vi "AlliGator Launcher.vi"() -> ()   [LabVIEW 2021, in "AlliGator GUI.lvlib"]
doc: "Runs transparently.\nLaunches AlliGator in transparent mode until initialization is complete."
uses:
  AlliGator GUI.lvlib
  AlliGator Variables List.ctl
  Notebook/Notebook Parameters List.ctl
  AlliGator Globals.vi
  AlliGator Check Version.vi
  Variant/Variant to Data/Variant to Boolean.vi
  <userlib>/_OpenG.lib/array/array.llb/Filter 1D Array (String)__ogtk.vi
  AlliGator Globals, Variables & Constants.lvlib
  Variant/Variant to Data/Variant to Data.lvlib
  Notebook/Notebook.lvlib
  Utilities/Utilities.lvlib
  AlliGator Action Engine.lvlib
  Error/Error.lvlib
  <userlib>/_OpenG.lib/array/array.llb/openg_array.lvlib
panel:
  out "About Message":string="© 2015-2023 The Regents of University of California\nAuthor: X. Michalet, Department of Chemistry & Biochemistry, UCLA\n\nThis software product was developed using LabVIEW™ and the National Instruments Vision Development Toolkit for LabVIEW. LabVIEW is a trademark of National Instruments.\n\nFunding was provided in part by grants from the US National Institute of Health, US Department of Energy, UC Cancer Research Coordination Committee and the UCLA Jonsson Comprehensive Cancer Center. AlliGator is not endorsed by, or sponsored by any of the above organizations.\n\nThis software is provided without guaranty of any kind, whether expressed or implied."
  out "Message":string
  out "Version":string
  out "Alligator":string="  AlliGator"
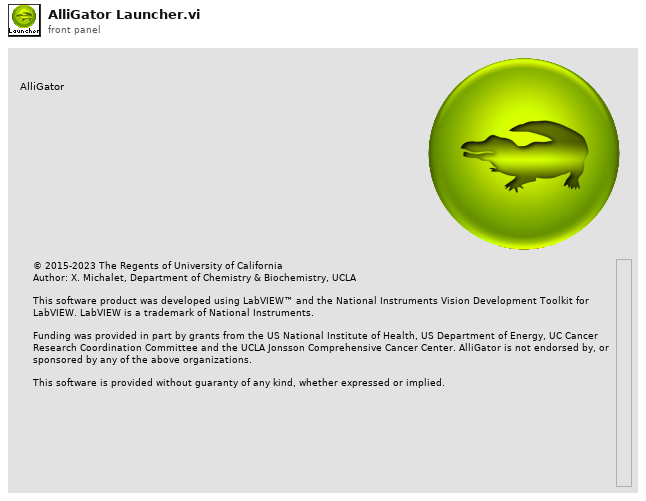
[diagram p1: front panel]
types:
  T1 = typedef "Notebook.lvlib/Notebook Parameters List.ctl" = enum16{"First Opening?", "Saved Notebook?", "Saved Notebook Path", "Beep on Error?"}
  T2 = enum32{"Invalid", "Standard", "Closed", "Hidden", "Minimized", "Maximized"}
  T3 = typedef "AlliGator Globals, Variables & Constants.lvlib/AlliGator Variables List.ctl" = enum16{"---- GUI ----", "Initialization Status", "State Indicators Refnum", "Original AlliGator Menu Items", "Current Action Loop State", "Script in progress", "Playback", "Loop Playback", "Search ROI Used", "Search ROI", "Decay Graph Max Legend Size", "Intensity Graph Max Legend Size", "Decay Statistics Graph Max Legend Size", "Phasor Graph Max Legend Size", "Phasor Ratio Graph Max Legend Size", "Lifetime Graph Max Legend Size", "---- Files ----", "Export Dataset Frames as Individual Files", "Show Batch Export Help Balloons", "Frames in Dataset", "ptu File Frame Start Indices", "Current Frame in Dataset", "Current Frame Timestamp", "------ Python Plugins ------", "Python Plugins Information", "Python Session", "Valid Python Session?", "---- Source Image ----", "Dataset Loaded", "Dataset Metadata", "Dataset Channel", "Dataset Data Description", "Background Dataset Metadata", "Background Dataset Channel", "Background Dataset Data Description", "Background File Subtraction", "Background File Path", "Background File Pile-up Correction", "Background File Pixel Well Capacity", "Background File Scaling Factor", "Source Image ROIs", "Current Source Image ROI", "Source Image ROI Event Refnum", "X_Source Image Display Range", "X_Source Image Palette Information", "Source Image Palette List", "Source Image Scale", "Current Dataset Load Settings", "Source Image:ROI Overlay Color", "---- Image Profile Window ----", "Image Profile:Overlay ROI in Source Image", "Image Profile Window Event Refnum", "Image Profile:IntensityType", "Image Profile:Intensity Average Type", "Image Profile:Intensity-weighted SDV", "Image Profile:Box Profile Type", "Image Profile Window Open", "Image Profile:Plotted Fit Parameter", "X_Type of Displayed Image", "X_Time Gate Slider", "Dataset Path", "Source Image Overlay to Erase", "Is Displayed Image Accumulated", "White Light Image Modified", "Mask Image Modified", "Macrotime Gate Separation", "------ Phasor Graph -------", "Phasor Graph:Show Line", "---- Phasor Plot ---", "Phasor Plot Parameters Changed", "FLI Dataset Modified since last Phasor Plot Calculation", "Phasor Harmonics Data", "Selected Phasor Harmonics", "Phasor Harmonic Manager Event Refnum", "Phasor Plot ROIs", "Current Phasor Plot ROI", "Phasor Plot ROI Event Refnum", "Phasor Plot Image Reference Points", "Phasor Plot Computed", "Phasor Plot Palette Information", "Phasor Plot Palette List", "Phasor Ratio Palette Information", "Phasor Ratio Palette List", "Phasor Image Scale", "Phasor Plot Image Overlay to Erase", "Phasor Plot Image Elements to Update", "Current Phasor Plot Calculation Parameters", "Current Phasor Calibration Options", "Reset Cumulated Phasor Plot", "Phasor Ratio Reference 1", "Phasor Ratio Lifetime Reference 1", "Phasor Ratio Reference 1 Frequency", "Phasor Ratio Reference 2", "Phasor Ratio Lifetime Reference 2", "Phasor Ratio Reference 2 Frequency", "---- Decay Analysis ----", "Number of Selected Decays to Fit", "LS Fit Results", "LAR Fit Results", "BS Fit Results", "Last Decay Max - Min", "Best Fit Parameters", "Best Fit Parameter Names", "Actual Size X", "Actual Size Y", "Binning X", "Binning Y", "Actual # Gates", "Dataset Number", "Gates to...", "Gates Skipped", "Gates to keep", "Gate Step", "Gate Separation", "Reversed Gates", "Pile-up Correction", "Pixel Well Capacity", "Background Subtracted", "Background Subtraction Method", "Background Definition Range", "Background File (deprecated)", "Number of Dataset Accumulated", "Array of Accumulated Dataset Paths", "Do Averaged Datasets", "Destination File Path", "Process Plot Target", "Use 1/D as Phasor Frequency", "---- Decay Fit Parameter Map -----", "Decay Fit Parameter Map Palette Information", "Decay Fit Parameter Map Palette List", "Local Decay Graph Window Event Refnum", "------- Local Decay Window ---------", "Use normalized IRF for convolution", "----- Miscellaneous ----", "Skippable Dialog Windows Status"}
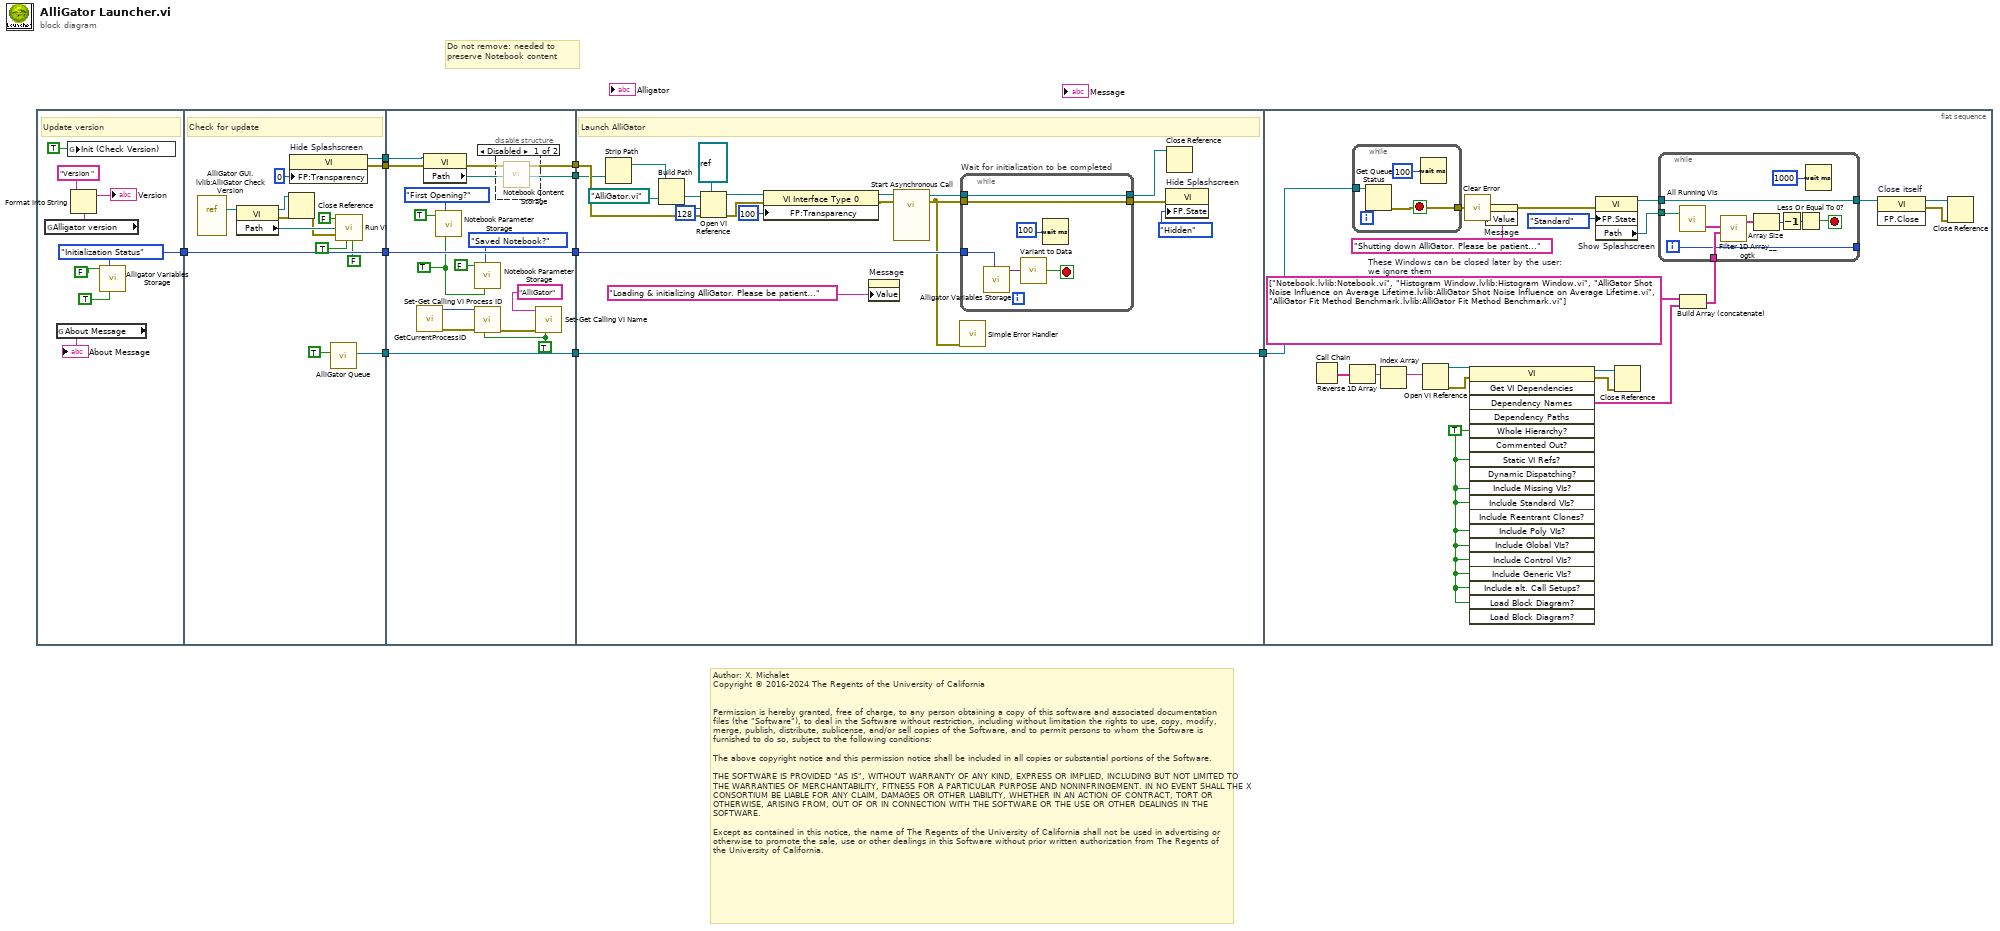
[diagram p0: block diagram]
diagram:
  # "Author: X. Michalet\nCopyright © 2016-2024 The Regents of the University of California\n \n\nPermission is hereby granted, free of charge, to any person obtaining a copy of this software and associated documentation files (the \"Software\"), to deal in the Software without restriction, including without limitation the rights to use, copy, modify, merge, publish, distribute, sublicense, and/or sell copies of the Software, and to permit persons to whom the Software is furnished to do so, subject to the following conditions:\n\nThe above copyright notice and this permission notice shall be included in all copies or substantial portions of the Software.\n\nTHE SOFTWARE IS PROVIDED \"AS IS\", WITHOUT WARRANTY OF ANY KIND, EXPRESS OR IMPLIED, INCLUDING BUT NOT LIMITED TO THE WARRANTIES OF MERCHANTABILITY, FITNESS FOR A PARTICULAR PURPOSE AND NONINFRINGEMENT. IN NO EVENT SHALL THE X CONSORTIUM BE LIABLE FOR ANY CLAIM, DAMAGES OR OTHER LIABILITY, WHETHER IN AN ACTION OF CONTRACT, TORT OR OTHERWISE, ARISING FROM, OUT OF OR IN CONNECTION WITH THE SOFTWARE OR THE USE OR OTHER DEALINGS IN THE SOFTWARE.\n\nExcept as contained in this notice, the name of The Regents of the University of California shall not be used in advertising or otherwise to promote the sale, use or other dealings in this Software without prior written authorization from The Regents of the University of California."
  # "Do not remove: needed to preserve Notebook content"
  n1 = flat-sequence {
    tunnel: [w15] -> w10
    tunnel: [w32] -> w9
    tunnel: w10 -> [w32]
    tunnel: [w30] -> w5
    tunnel: [w29] -> w4
    tunnel: [w28] -> w3
    tunnel: w9 -> [w48]
    tunnel: [w48] -> w8
    tunnel: [w42] -> w6
    tunnel: w5 -> [w42]
    tunnel: w4 -> [w41]
    tunnel: w3 -> [w40]
    tunnel: [w39] -> w2
    tunnel: [w38] -> w1
    tunnel: w8 -> [w63]
    tunnel: [w53] -> w7
    tunnel: w6 -> [w53]
    tunnel: w2 -> [w51]
    tunnel: w1 -> [w50]
    tunnel: w7 -> [w91]
    frame #0 {
      w15 = AlliGator_Variables_List."Initialization Status" ("Alligator Variable")
      # "Update version"
      n2 = global read "AlliGator Globals.vi" "Alligator version"() -> (w12:string)
      n3 = global read "AlliGator Globals.vi" "About Message"() -> (→"About Message":string)
      n4 = global write "AlliGator Globals.vi" "Init (Check Version)"(TRUE ("Init (Check Version)")) -> ()
      n5 = Format Into String(initial string="Version ", w12) -> (resulting string=→"Version":string)  [unwired: 2 in, 1 out]
      n6 = call "Alligator Variables Storage.vi"("Get(F)/Set"=TRUE, "AlliGator Variable"=w15, "Data in"=FALSE ("Get(F)/Set")) -> ()  [unwired: 6 in, 3 out]
    }
    frame #1 {
      # "Check for update"
      n7 = vi-ref "AlliGator GUI.lvlib:AlliGator Check Version.vi"() -> (w27:refnum<vi>)
      n8 = property class="VI"(reference=w27) -> (reference out=w22:refnum<vi>, error out=w21:errorcluster, "Path"=w26:path)  [unwired: 1 in]
      n9 = Close Reference(reference=w22, error in (no error)=w21) -> (error out=w20:errorcluster)
      n10 = property on="Hide Splashscreen" class="VI"("FP:Transparency"=u8 0 ("Front Panel Window:Transparency")) -> (reference out=w29:refnum<vi>, error out=w28:errorcluster)  [unwired: 2 in]
      n11 = call "AlliGator Queue.vi"("create if not found? (F)"=TRUE) -> ("AlliGator Queue"=w30:refnum<queue>)  [unwired: 7 in, 1 out]
      n12 = call "Run Vi.vi"("Bring To Front (T)"=FALSE, "VI Path"=w26, "error in (no error)"=w20, "Start Hidden? (F)"=TRUE, "Activate? (T)"=FALSE) -> ()  [unwired: 3 in, 2 out]
    }
    frame #2 {
      w33 = TRUE ("Get(F)/Set")
      w44 = TRUE ("Set/Get (F)")
      n13 = call "GetCurrentProcessID.vi"() -> ("Error Out"=w47:errorcluster, "ProcessID"=w46:u32)  [unwired: 10 in]
      n14 = property class="VI"(reference=w41, error in=w40) -> (error out=w39:errorcluster, "Path"=w38:path)  [unwired: 1 out]
      n15 = call "Notebook Parameter Storage.vi"("Get(F)/Set"=w33, "Notebook Parameter List"=Notebook_Parameters_List."First Opening?", "Data in"=TRUE ("Start Hidden? (F)")) -> ()  [unwired: 7 in, 2 out]
      n16 = call "Notebook Parameter Storage.vi"("Get(F)/Set"=w33, "Notebook Parameter List"=Notebook_Parameters_List."Saved Notebook?", "Data in"=FALSE ("Saved Notebook?")) -> ()  [unwired: 7 in, 2 out]
      n17 = call "Set-Get Calling VI Process ID.vi"("Set/Get (F)"=w44, "Error In"=w47, "ProcessID"=w46) -> ("Error Out"=w45:errorcluster)  [unwired: 7 in, 1 out]
      n18 = disable-structure shown="Disabled" {
        frame Disabled {
          n19 = call "Notebook Content Storage.vi"() -> ()  [unwired: 10 in, 2 out]
        }
        frame Enabled {
        }
      }
      n20 = call "Set-Get Calling VI Name.vi"("Set/Get (F)"=w44, "Error In"=w45, "Calling VI Name"="AlliGator" ("Main VI Name")) -> ()  [unwired: 7 in, 2 out]
    }
    frame #3 {
      # "Launch AlliGator"
      n21 = Strip Path(path=w50) -> (stripped path=w49:path)  [unwired: 1 out]
      n22 = Build Path(base path=w49, name or relative path=path "AlliGator.vi" ("vi path")) -> (appended path=w52:path)
      n23 = Open VI Reference(type specifier VI Refnum (for type only)=refnum<vi> refnum, vi path=w52, options=128, error in (no error)=w51) -> (vi reference=w57:refnum<vi>, error out=w56:errorcluster)  [unwired: 2 in]
      n24 = property class="VI Interface Type 0"(reference=w57, error in=w56, "FP:Transparency"=u8 100 ("Front Panel Window:Transparency")) -> (reference out=w55:refnum<vi>, error out=w54:errorcluster)
      n25 = property on="Message" class="Str"("Value"="Loading & initializing AlliGator. Please be patient..." ("Message")) -> ()  [unwired: 2 in, 2 out]
      n26 = call-by-ref "Start Asynchronous Call"(reference=w55, error in=w54) -> (reference out=w67:refnum<vi>, error out=w61:errorcluster)  [unwired: 1 in]
      n27 = call <vilib>:"Simple Error Handler.vi"("error in (no error)"=w61) -> ()  [unwired: 4 in, 5 out]
      n28 = while "Wait for initialization to be completed" {
        tunnel: w67 -> [w73]
        tunnel: w61 -> [w72]
        tunnel: [w73] -> w62
        tunnel: [w72] -> w64
        tunnel: w63 -> [w71]
        stop <- w69 stop-if-true
        n29 = call "Alligator Variables Storage.vi"("AlliGator Variable"=w71) -> ("Data out"=w70:variant)  [unwired: 8 in, 2 out]
        n30 = call-poly "Variant to Data.vi"("Variant"=w70) -> ("Value"=w69:bool)  [unwired: 8 in]
        n31 = Wait (ms)(milliseconds to wait=u32 100) -> ()  [unwired: 1 out]
      }
      n32 = property on="Hide Splashscreen" class="VI"(error in=w64, "FP.State"=T2."Hidden" ("Front Panel Window:State")) -> ()  [unwired: 1 in, 2 out]
      n33 = Close Reference(reference=w62) -> ()  [unwired: 1 in, 1 out]
    }
    frame #4 {
      w89 = string[] ["Notebook.lvlib:Notebook.vi", "Histogram Window.lvlib:Histogram Window.vi", "AlliGator Shot Noise Influence on Average Lifetime.lvlib:AlliGator Shot Noise Influence on Average Lifetime.vi", "AlliGator Fit Method Benchmark.lvlib:AlliGator Fit Method Benchmark.vi"]  # These Windows can be closed later by the user: we ignore them
      w77 = TRUE ("Whole Hierarchy?")
      n34 = Call Chain() -> (call chain=w84:string[])
      n35 = Reverse 1D Array(array=w84) -> (reversed array=w83:string[])
      n36 = while {
        tunnel: w91 -> [w109]
        tunnel: [w108] -> w85
        stop <- w108 stop-if-true
        n37 = Get Queue Status(queue=w109) -> (error out=w108:errorcluster)  [unwired: 2 in, 7 out]
        n38 = Wait (ms)(milliseconds to wait=u32 100) -> ()  [unwired: 1 out]
      }
      n39 = Index Array(array=w83) -> (element=w82:string)  [unwired: 1 in]
      n40 = Open VI Reference(vi path=w82) -> (vi reference=w81:refnum<vi>, error out=w80:errorcluster)  [unwired: 5 in]
      n41 = call "Clear Error.vi"("Error In"=w85) -> ("no Error Out"=w90:errorcluster)  [unwired: 8 in]
      n42 = invoke class="VI" method="Get VI Dependencies"(reference=w81, error in=w80, "Whole Hierarchy?"=w77, "Static VI Refs?"=w77, "Include Missing VIs?"=w77, "Include Standard VIs?"=w77, "Include Poly VIs?"=w77, "Include Global VIs?"=w77, "Include Control VIs?"=w77, "Include Generic VIs?"=w77, "Include alt. Call Setups?"=w77, "Load Block Diagram?"=w77) -> (reference out=w76:refnum<vi>, error out=w75:errorcluster, "Dependency Names"=w78:string[])  [unwired: 7 in, 16 out]
      n43 = property on="Message" class="Str"(error in=w90, "Value"="Shutting down AlliGator. Please be patient..." ("Message")) -> (error out=w94:errorcluster)  [unwired: 1 in, 1 out]
      n44 = property on="Show Splashscreen" class="VI"(error in=w94, "FP.State"=T2."Standard" ("Front Panel Window:State")) -> (reference out=w88:refnum<vi>, "Path"=w86:path)  [unwired: 1 in, 1 out]
      n45 = Close Reference(reference=w76, error in (no error)=w75) -> ()  [unwired: 1 out]
      n46 = Build Array (concatenate)(w89, w78) -> (w79:string[])
      n47 = while {
        tunnel: w79 -> [w105]
        tunnel: w88 -> [w100]
        tunnel: [w100] -> w87
        tunnel: w86 -> [w99]
        tunnel: [w97] -> _
        i -> [w97]
        stop <- w101 stop-if-true
        n48 = call "All Running Vis.vi"("Calling Vi path"=w99) -> ("Runnning Vi Names"=w106:string[])  [unwired: 1 in, 1 out]
        n49 = call-poly <userlib>:"Filter 1D Array__ogtk.vi"("items to filter"=w105, "array"=w106) -> ("filtered array"=w104:string[])  [unwired: 4 in, 1 out]
        n50 = Array Size(array=w104) -> (size(s)=w103:i32)
        n51 = Decrement(x=w103) -> (x-1=w102:i32)
        n52 = Less Or Equal To 0?(x=w102) -> (x <= 0?=w101:bool)
        n53 = Wait (ms)(milliseconds to wait=u32 1000) -> ()  [unwired: 1 out]
      }
      n54 = invoke on="Close itself" class="VI" method="FP.Close"(reference=w87) -> (reference out=w95:refnum<vi>, error out=w96:errorcluster)  [unwired: 2 in, 1 out]
      n55 = Close Reference(reference=w95, error in (no error)=w96) -> ()  [unwired: 1 out]
    }
  }
